vi "GoalKickKeeperTacticCheckStateChange.vi"(8 "error in (no error)":errorcluster, 9 "Game in":refnum<class "Game.lvclass">, 10 "Robot In":refnum<class "Robot.lvclass">, 11 "GoalKickKeeperTacticVSS in":refnum<class "GoalKickKeeperTacticVSS.lvclass">) -> (0 "error out":errorcluster, 2 "States":enum16{"GoToBallKeeper", "Kick", "Exit"}(ring), 3 "GoalKickKeeperTacticVSS out":refnum<class "GoalKickKeeperTacticVSS.lvclass">)   [LabVIEW 2020, in "GoalKickKeeperTacticVSS.lvclass"]
uses:
  GoalKickKeeperTacticVSS.lvclass
  Robot_class/Robot.lvclass
  Game_class/Game.lvclass
  Game_class/Game.lvclass/Game.ctl
  Utilities_class/Utilities.lvclass
  Game_class/Read BallRef.vi
  Ball_class/Ball.lvclass
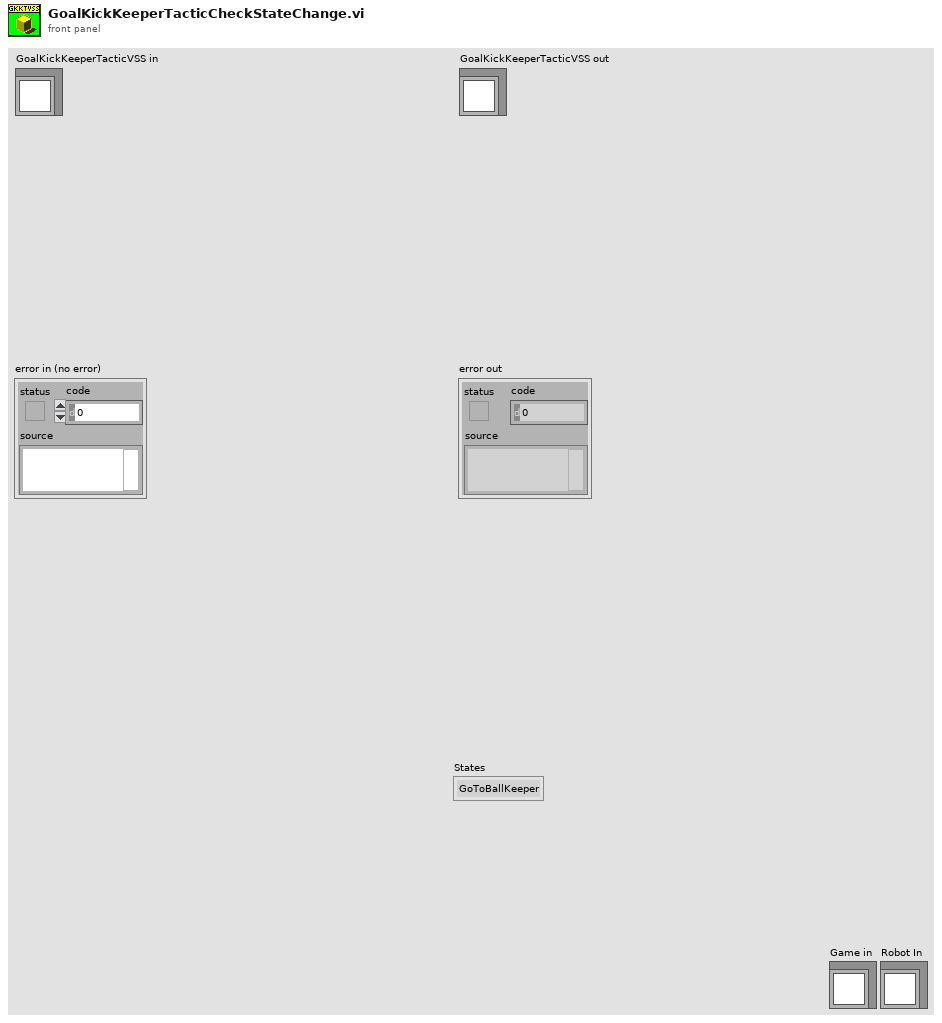
[diagram p1: front panel]
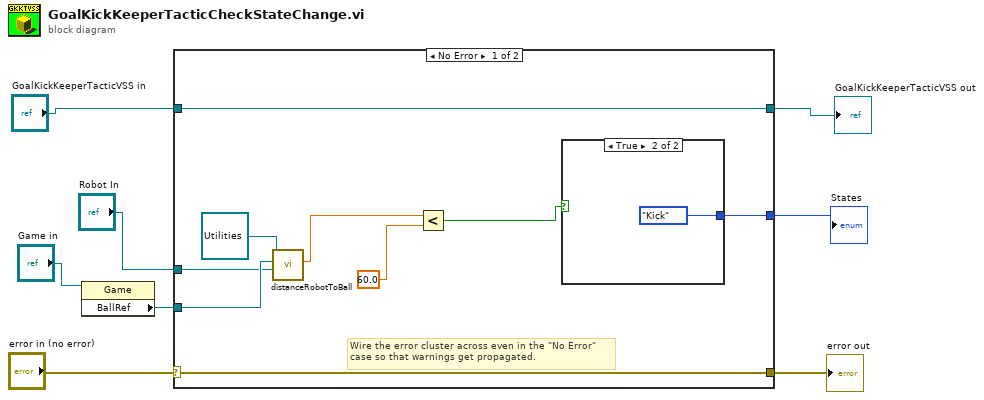
[diagram p0: block diagram]
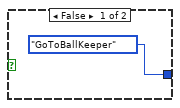
[diagram p2: hidden frame]
diagram:
  n1 = property class="Game"(reference="Game in") -> ("BallRef"=w6:refnum<class "Ball.lvclass">)  [unwired: 1 in, 2 out]
  n2 = case shown="No Error" "error in (no error)" {
    selector: "error in (no error)" -> [w16 w21]
    tunnel: [w16 w21] -> w4
    tunnel: [w17 w20] -> w1
    tunnel: "GoalKickKeeperTacticVSS in" -> [w17 w20]
    tunnel: [w15 _] -> w8
    tunnel: w6 -> [w10 _]
    tunnel: "Robot In" -> [w9 _]
    frame No Error {
      # "Wire the error cluster across even in the \"No Error\"\ncase so that warnings get propagated."
      n3 = call "distanceRobotToBall.vi"("Robot"=w9, "Ball"=w10, "Utilities in"=refnum<class "Utilities.lvclass"> refnum) -> ("Distance Robot To Ball"=w13:dbl)  [unwired: 6 in, 2 out]
      n4 = Less?(x=w13, y=60.0) -> (x < y?=w11:bool)
      n5 = case shown="True" w11 {
        tunnel: [enum16{"GoToBallKeeper", "Kick", "Exit"}."GoToBallKeeper" ("State") enum16{"GoToBallKeeper", "Kick", "Exit"}."Kick" ("State")] -> w15
        frame False {
        }
        frame True {
        }
      }
    }
    frame Error {
    }
  }
  "error out" <- w4
  "GoalKickKeeperTacticVSS out" <- w1
  "States" <- w8
